vi "Laser Control.vi"(8 "error in (no error)":errorcluster, 10 "Laser 2":bool, 11 "Laser 1":bool) -> (0 "error out":errorcluster)   [LabVIEW 2015, in "Tool Interface.lvlib"]
uses:
  Tool Interface.lvlib
  Tool Typedefs/_Laser Ctrl Cluster--typedef.ctl
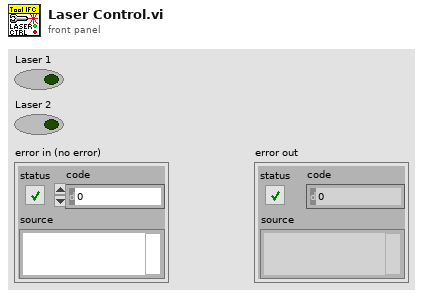
[diagram p1: front panel]
types:
  T1 = typedef "_Laser Ctrl Cluster--typedef.ctl" = cluster{"Laser 1":bool, "Laser 2":bool}
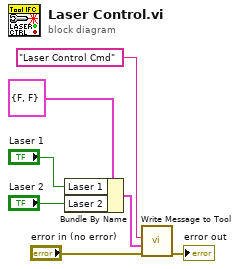
[diagram p0: block diagram]
diagram:
  n1 = Bundle By Name(cluster=T1 {"Laser 1"=FALSE, "Laser 2"=FALSE} ("_Set Laser Params Cluster--typedef"), "Laser 1"="Laser 1", "Laser 2"="Laser 2") -> (w6:T1)
  n2 = call "Write Message to Tool.vi"("error in (no error)"="error in (no error)", "Message Data"=w6, "Message"="Laser Control Cmd") -> ("error out"=→"error out":errorcluster)  [unwired: 8 in]
